vi "DAQ.44xx.Get AO Min and Max.vi"(8 "error in (no error)":errorcluster, 9 "AO.channels":tag, 10 "AO.Range":T1) -> (0 "error out":errorcluster, 1 "AO.channels out":tag, 2 "AO.max":dbl, 3 "AO.min":dbl)   [LabVIEW 2019, in "Instrument.Lockin.lvlib" / "Instrument.DAQ.lvclass"]
uses:
  Instrument.DAQ.lvclass
  Typedefs/DAQ.Config.AO.Range--enum.ctl
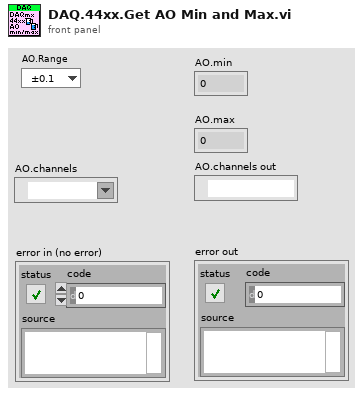
[diagram p1: front panel]
types:
  T1 = typedef "Instrument.Lockin.lvlib/Instrument.DAQ.lvclass/DAQ.Config.AO.Range--enum.ctl" = enum16{"±0.1", "±1.0", "±10.0", ""}
  T2 = typedef "Instrument.Lockin.lvlib/Instrument.DAQ.lvclass/DAQ.Type--enum.ctl" = enum16{"None", "USB-4431", "PXI-446x"}
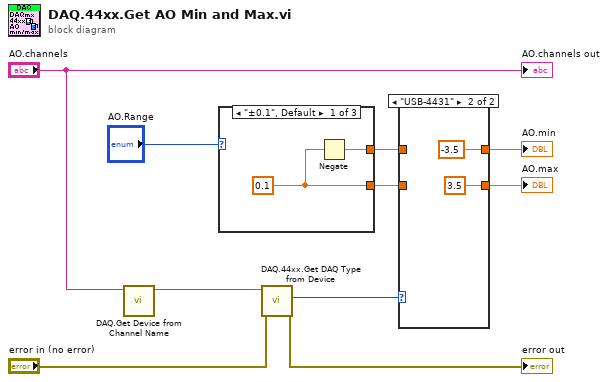
[diagram p0: block diagram]
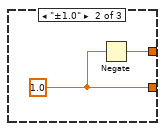
[diagram p2: hidden frame]
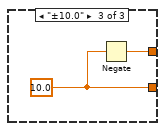
[diagram p3: hidden frame]
diagram:
  n1 = call "DAQ.Get Device from Channel Name.vi"("Channel"="AO.channels") -> ("Device"=w1:tag)  [unwired: 10 in]
  n2 = case shown="\"±0.1\", Default" "AO.Range" {
    tunnel: [w12 w14 w16] -> w6
    tunnel: [w11 w13 w15] -> w8
    frame "±0.1", Default {
      w12 = 0.1
      n3 = Negate(x=w12) -> (-x=w11:dbl)
    }
    frame "±1.0" {
      w14 = 1.0
      n4 = Negate(x=w14) -> (-x=w13:dbl)
    }
    frame "±10.0" {
      w16 = 10.0
      n5 = Negate(x=w16) -> (-x=w15:dbl)
    }
  }
  n6 = call "DAQ.44xx.Get DAQ Type from Device.vi"("error in (no error)"="error in (no error)", "DAQmx Device Name"=w1) -> ("error out"=→"error out":errorcluster, "DAQ Type"=w5:T2)  [unwired: 7 in, 1 out]
  n7 = case shown="\"USB-4431\"" w5 {
    tunnel: [w18 -3.5] -> w9
    tunnel: w8 -> [w18 _]
    tunnel: [w17 3.5] -> w7
    tunnel: w6 -> [w17 _]
    frame Default {
    }
    frame "USB-4431" {
    }
  }
  "AO.min" <- w9
  "AO.max" <- w7
  "AO.channels out" <- "AO.channels"
